vi "Add System Mappings.vi"(8 "error in (no error)":errorcluster, 9 "Settings":T1, 11 "SysDef Ref":T3) -> (0 "error out":errorcluster, 3 "SysDef Ref Out":T3)   [LabVIEW 2019, in "Simple SysDef API.lvlib"]
uses:
  <userlib>/SimpleSysDef/Simple SysDef API.lvlib
  <userlib>/SimpleSysDef/_SubVIs/System Definition Reference.ctl
  NationalInstruments.VeriStand.SystemDefinitionAPI
  <userlib>/SimpleSysDef/_SubVIs/Add System Mappings_Settings.ctl
  <userlib>/SimpleSysDef/_SubVIs/Add System Mappings_Settings_Channel Pairs.ctl
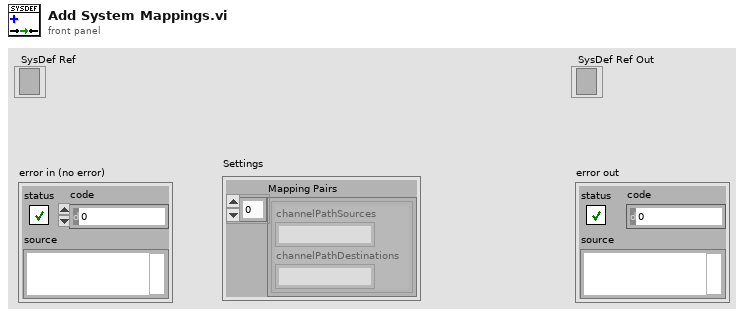
[diagram p1: front panel]
types:
  T1 = typedef "Simple SysDef API.lvlib/Add System Mappings_Settings.ctl" = cluster{"Mapping Pairs":T2[]}
  T2 = typedef "Simple SysDef API.lvlib/Add System Mappings_Settings_Channel Pairs.ctl" = cluster{"channelPathSources":string, "channelPathDestinations":string}
  T3 = typedef "Simple SysDef API.lvlib/System Definition Reference.ctl" = refnum<k24>
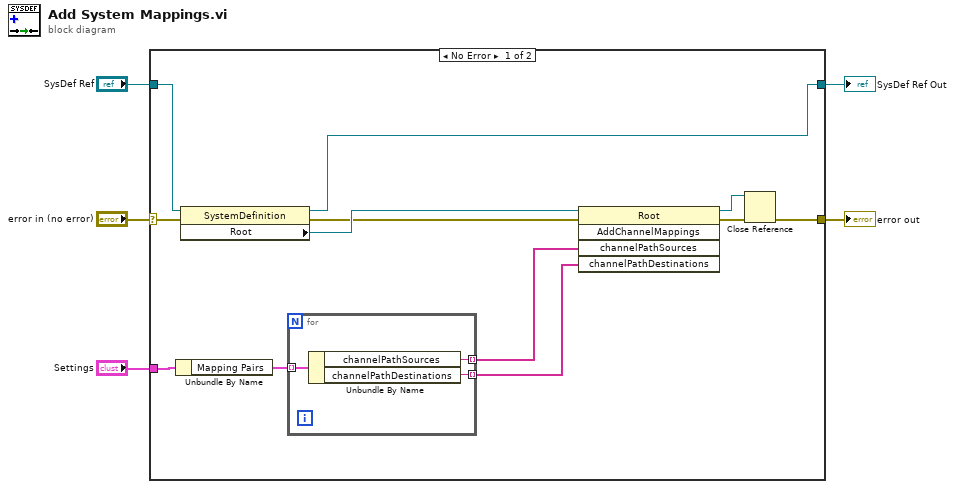
[diagram p0: block diagram]
diagram:
  n1 = case shown="No Error" "error in (no error)" {
    selector: "error in (no error)" -> [w15 w22]
    tunnel: [w16 w22] -> w4
    tunnel: "SysDef Ref" -> [w14 w21]
    tunnel: [w13 w21] -> w2
    tunnel: "Settings" -> [w17 _]
    frame No Error {
      n2 = Unbundle By Name(w17) -> ("Mapping Pairs"=w8:T2[])
      n3 = property class="SystemDefinition"(reference=w14, error in=w15) -> (reference out=w13:T3, error out=w11:errorcluster, "Root"=w12:refnum<k24>)
      n4 = for {
        tunnel: w8 -> [w20] mode=indexing
        tunnel: [w19] -> w7 mode=indexing
        tunnel: [w18] -> w6 mode=indexing
        n5 = Unbundle By Name(w20) -> ("channelPathSources"=w19:string, "channelPathDestinations"=w18:string)
      }
      n6 = invoke class="Root" method="AddChannelMappings"(reference=w12, error in=w11, "channelPathSources"=w7, "channelPathDestinations"=w6) -> (reference out=w9:refnum<k24>, error out=w10:errorcluster)  [unwired: 1 in, 3 out]
      n7 = Close Reference(reference=w9, error in (no error)=w10) -> (error out=w16:errorcluster)
    }
    frame Error {
    }
  }
  "SysDef Ref Out" <- w2
  "error out" <- w4
